vi "Event Adaptive Size.vi"(8 "error in (no error)":errorcluster, 11 "Normal Log in":refnum<class "Normal Log.lvclass">) -> (0 "error out":errorcluster, 3 "Normal Log out":refnum<class "Normal Log.lvclass">)   [LabVIEW 2020, in "Normal Log.lvlib" / "Normal Log.lvclass"]
uses:
  Normal Log.lvclass
  <vilib>/Utility/miscctls.llb/LVRowAndColumnTypeDef.ctl
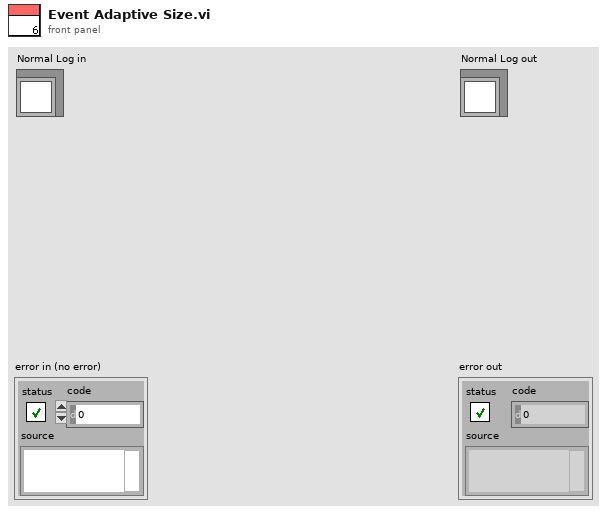
[diagram p1: front panel]
types:
  T1 = typedef "LVRowAndColumnTypeDef.ctl" = cluster{"Row":i32, "Column":i32}
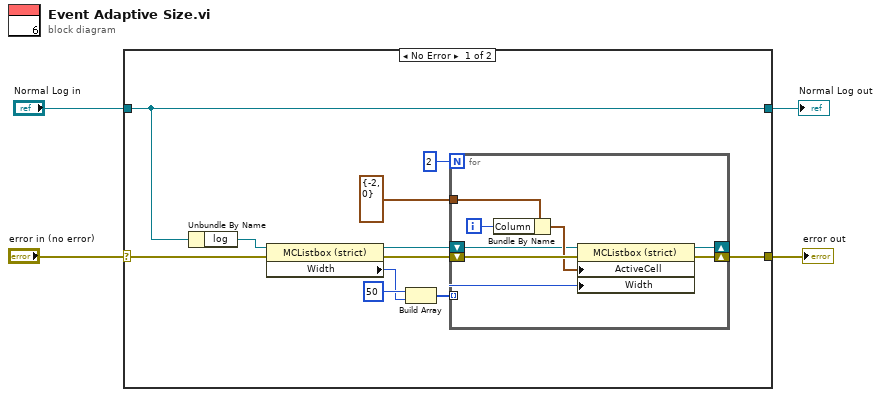
[diagram p0: block diagram]
diagram:
  n1 = case shown="No Error" "error in (no error)" {
    selector: "error in (no error)" -> [w6 w25]
    tunnel: [w5 w25] -> w1
    tunnel: [w7 w24] -> w2
    tunnel: "Normal Log in" -> [w7 w24]
    frame No Error {
      n2 = Unbundle By Name(w7) -> ("log"=w8:refnum<vi>)
      n3 = property on="Property Node" class="MCListbox (strict)"(reference=w8, error in=w6) -> (reference out=w9:refnum<vi>, error out=w15:errorcluster, "Width"=w13:u32)
      n4 = Build Array(50, w13) -> (w12:u32[])
      n5 = for {
        N: 2 -> [_]
        shift-right: [w22] -> w5
        shift-left: w15 -> [w23]
        tunnel: w12 -> [w21] mode=indexing
        tunnel: T1 {"Row"=-2, "Column"=0} ("Active Cell:Active Cell") -> [w20]
        shift-right: [w16] -> _
        shift-left: w9 -> [w17]
        i -> [w19]
        n6 = Bundle By Name(cluster=w20, "Column"=w19) -> (w18:T1)
        n7 = property on="Property Node" class="MCListbox (strict)"(reference=w17, error in=w23, "ActiveCell"=w18, "Width"=w21) -> (reference out=w16:refnum<vi>, error out=w22:errorcluster)
      }
    }
    frame Error {
    }
  }
  "error out" <- w1
  "Normal Log out" <- w2
